vi "IR Transmit NEC.vi"(8 "Error In":errorcluster, 9 "Data":u8=52, 10 "Address":u8=52, 11 "Arduino Resource":T1={"VISA resource"="", "Board Type"=enum."Arduino Uno", "Connection Type"=enum."USB / Serial", "Bytes Per Packet (15)"=15}) -> (0 "Error Out":errorcluster, 3 "Arduino Resource":T1={"VISA resource"="", "Board Type"=enum."Arduino Uno", "Connection Type"=enum."USB / Serial", "Bytes Per Packet (15)"=15})   [LabVIEW 2011, in "LabVIEW Interface for ChipKit.lvlib"]
uses:
  LabVIEW Interface for ChipKit.lvlib
  Private/Type Defs/Chipkit Resource.ctl
  Private/Type Defs/Board Type.ctl
  Private/Type Defs/IR Type.ctl
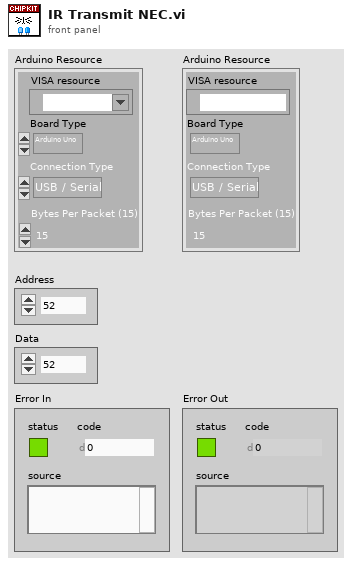
[diagram p1: front panel]
types:
  T1 = typedef "LabVIEW Interface for ChipKit.lvlib/Chipkit Resource.ctl" = cluster{"VISA resource":refnum<visa-resource-name>, "Board Type":T2, "Connection Type":enum8{"USB / Serial"}, "Bytes Per Packet (15)":u8}
  T2 = typedef "LabVIEW Interface for ChipKit.lvlib/Board Type.ctl" = enum16{"Arduino Uno", "Dimuelanove w/Atmega 328", "Mega 2560", "Chipkit Uno32", "Chipkit Max32"}
  T3 = typedef "LabVIEW Interface for ChipKit.lvlib/IR Type.ctl" = enum8{"NEC", "Sony", "RC5", "RC6"}
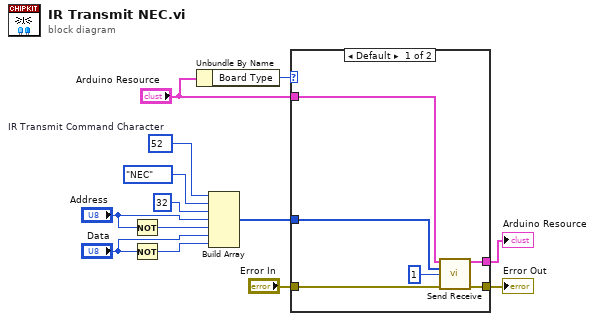
[diagram p0: block diagram]
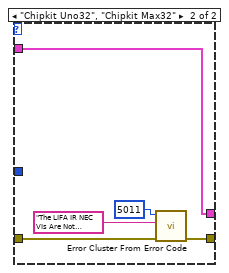
[diagram p2: hidden frame]
diagram:
  w8 = u8 52  # IR Transmit Command Character
  n1 = Not(x="Address") -> (.not. x?=w11:u8)
  n2 = Not(x="Data") -> (.not. x?=w9:u8)
  n3 = Unbundle By Name("Arduino Resource") -> ("Board Type"=w4:T2)
  n4 = Build Array(w8, IR_Type."NEC" ("IR Type"), u8 32 ("element"), "Address", w11, "Data", w9) -> (w2:u8[])
  n5 = case shown="Default" w4 {
    tunnel: "Error In" -> [w18 w22]
    tunnel: [w16 w21] -> w1
    tunnel: "Arduino Resource" -> [w17 w20]
    tunnel: w2 -> [w15 _]
    tunnel: [w14 w20] -> w3
    frame Default {
      n6 = call "Send Receive.vi"("Arduino Resource"=w17, "Data"=w15, "Bytes To Read (0)"=u8 1, "error in"=w18) -> ("Arduino Resource"=w14:T1, "error out"=w16:errorcluster)  [unwired: 9 in, 1 out]
    }
    frame "Chipkit Uno32", "Chipkit Max32" {
      n7 = call <vilib>:"Error Cluster From Error Code.vi"("error in (no error)"=w22, "error message (\"\")"="The LIFA IR NEC VIs Are Not Supported On Chipkit Targets." ("source"), "error code (0)"=5011) -> ("error out"=w21:errorcluster)  [unwired: 6 in]
    }
  }
  "Arduino Resource" <- w3
  "Error Out" <- w1
